vi "x-axis.vi"(8 "error in (no error)":errorcluster, 11 "Wavelength PEM and Digikröm in":refnum<class "Wavelength PEM and Digikröm.lvclass">) -> (0 "error out":errorcluster, 1 "Label":string, 2 "Unit":string, 3 "Wavelength PEM and Digikröm out":refnum<class "Wavelength PEM and Digikröm.lvclass">)   [LabVIEW 2023, in "Wavelength PEM and Digikröm.lvclass"]
uses:
  Scanner/Scanner.lvclass
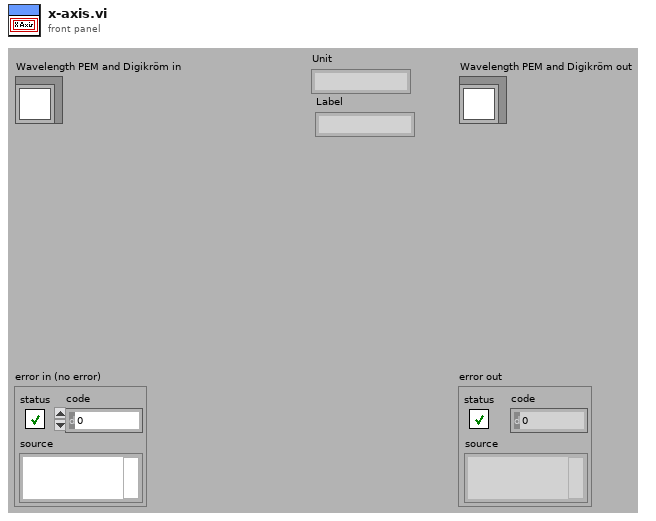
[diagram p1: front panel]
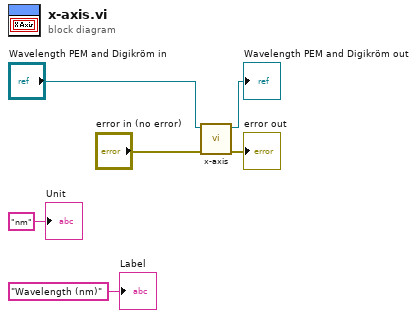
[diagram p0: block diagram]
diagram:
  n1 = call-parent "x-axis.vi"("error in (no error)"="error in (no error)", "Scanner in"="Wavelength PEM and Digikröm in") -> ("error out"=→"error out":errorcluster, "Scanner out"=→"Wavelength PEM and Digikröm out":refnum<class "Wavelength PEM and Digikröm.lvclass">)  [unwired: 6 in, 2 out]
  "Label" <- "Wavelength (nm)" ("Label")
  "Unit" <- "nm" ("Unit")
